vi "Vol-RPM_Tuning.vi"() -> ()   [LabVIEW 2014]
uses:
  LabView/PXI_Interface/AnalogInput/AnalogInput.lvclass
  Classes/DataLogger/Data Logger.lvclass
  <vilib>/Platform/TimedLoop/XDataNode/timing_clust.ctl
  <vilib>/Platform/TimedLoop/XDataNode/nitl_modes.ctl
  <vilib>/Platform/TimedLoop/XDataNode/wakeup.ctl
  <vilib>/FPGAPlugInAG/PXI-7842R/niLvFpga_Open_PXI-7842R.vi
  <vilib>/rvi/interface/common/dynamic/niFpgaDynamicAddResources.vi
  <vilib>/FPGAPlugInAG/Dynamic/niLvFpga_Reset_Dynamic.vi
  <vilib>/FPGAPlugInAG/Dynamic/niLvFpga_Run_Dynamic.vi
  <vilib>/Utility/error.llb/Error Cluster From Error Code.vi
  <vilib>/rvi/errors/niLvFpgaAdjustHostInterfaceError.vi
  <vilib>/addons/control/pid/pid.llb/PID Control Input Filter (DBL).vi
  <vilib>/addons/control/pid/pid.llb/PID Advanced (DBL).vi
  <vilib>/addons/control/pid/pid.llb/PID Output Rate Limiter (DBL).vi
  <vilib>/rvi/interface/nirviOpenFPGA/nirviOpenFPGA.xnode
  FPGA Bitfiles/CAlex2_FPGATarget2_MotorControl_XW+iUkbXN4U.lvbitx
  FPGA2 VIs/MotorControl_PWM+AO.vi
  <vilib>/rvi/interface/nirviMethod/nirviMethod.xnode
  <vilib>/rvi/interface/nirviReadWriteControl/nirviReadWriteControl.xnode
  <vilib>/Platform/TimedLoop/XDataNode/XDataNode.xnode
  <vilib>/Platform/TimedLoop/XDataNode/XDNodeRunTimeDep.lvlib
  <vilib>/rvi/interface/Simulation/niFpgaSimulationCallBeginRW.vi
  <vilib>/addons/control/pid/NI_PID_pid.lvlib
  Classes/MotorControl/MotorControl.lvclass
  NiFpgaLv.dll
panel:
  out "Force (N)":dbl
  in  "Enum":enum16{"1", "2", "3", "4", "5", "6", "7", "8"}(ring)
  in  "Vfb":i32=8
  out "Current(A)":dbl
  in  "Vrpm":i32=9
  out "Speed(rpm)":dbl
  in  "File Name":string
  in  "End":dbl
  in  "Begin":dbl
  in  "Start":bool
  in  "Step":dbl
  in  "Duration":dbl
  out "Current":cluster{"output":dbl}(graph)
  in  "RateLimiter":dbl=1.0 format="%.2f"
  in  "PID":bool=TRUE
  in  "Manual AO":dbl format="%.2f"
  out "Angular Rates (RPM)":dbl[](array[numeric])
  in  "AO":dbl[](array[numeric])
  in  "Zero":bool
  out "Speed":T1(graph)
  in  "setpoint":dbl format="%.2f"
  in  "reinitialize? (F)":bool
  in  "PID gains":T2={"proportional gain (Kc)"=1.0, "integral time (Ti, min)"=0.01, "derivative time (Td, min)"=0.0} {"derivative time (Td, min)" format="%.5f"; "integral time (Ti, min)" format="%.5f"; "proportional gain (Kc)" format="%.5f"}
  in  "output range":cluster{"output high":dbl, "output low":dbl}={"output high"=5.0, "output low"=-5.0} {"output low" format="%.2f"; "output high" format="%.2f"}
  in  "AO Channel":enum16{"1", "2", "3", "4", "5", "6", "7", "8"}(ring)
  in  "Encoder Channel":T3(ring)
  out "AO Value":dbl[](array[numeric]) format="%.3f"
  in  "stop":bool
  out "Angles (deg)":dbl[](array[numeric])
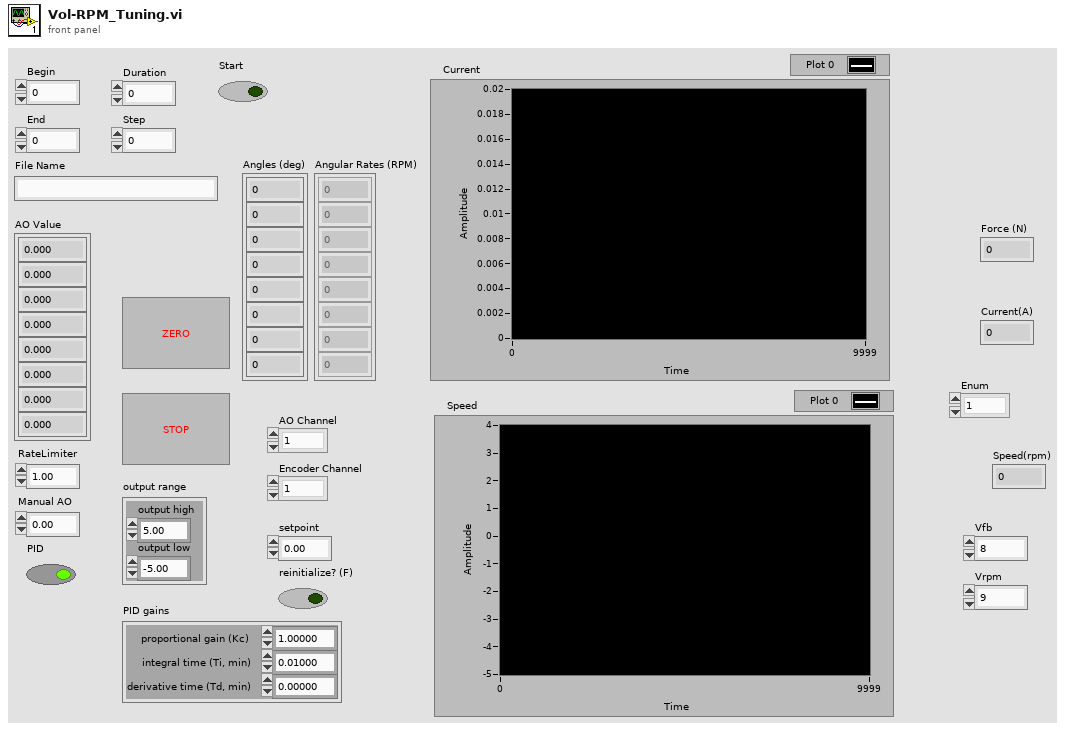
[diagram p1: front panel]
types:
  T1 = cluster{"setpoint":dbl, "output":dbl, "Speed(rpm)":dbl}
  T2 = cluster{"proportional gain (Kc)":dbl, "integral time (Ti, min)":dbl, "derivative time (Td, min)":dbl}
  T3 = enum16{"1", "2", "3", "4", "5", "6", "7", "8", "Vfb"}
  T4 = typedef "XDNodeRunTimeDep.lvlib/timing_clust.ctl" = cluster{"Expected End [f-1]":u64, "Actual End [f-1]":u64, "Finished Late? [f-1]":bool, "Expected End [i-1]":u64, "Actual End [i-1]":u64, "Finished Late? [i-1]":bool, "Expected Start [i]":u64, "Actual Start [i]":u64, "Expected Start [f]":u64, "Actual Start [f]":u64, "Source Name":string, "Structure Name":string, "Period":i64, "Deadline":i64, "Offset":i64, "Start":i64, "Priority":i32, "Timeout":i32, "Mode":T5, "Wakeup Reason":T6, "Error":errorcluster, "Source Type":string, "Secondary Source Type":string, "Global End Time":u64, "Global Start Time":u64, "Frame Duration":u64, "Iteration Duration":u64, "Assigned CPU":i32, "I/O Scan Engine Mode":u32}
  T5 = typedef "XDNodeRunTimeDep.lvlib/nitl_modes.ctl" = enum32{"No Change", "Process missed periods, maintain original phase", "Discard missed periods, maintain original phase", "Process missed periods, ignore original phase", "Discard missed periods, ignore original phase"}
  T6 = typedef "XDNodeRunTimeDep.lvlib/wakeup.ctl" = enum32{"Normal", "Aborted", "Asynchronous wakeup", "Timing source error", "Timed loop error", "Timeout"}
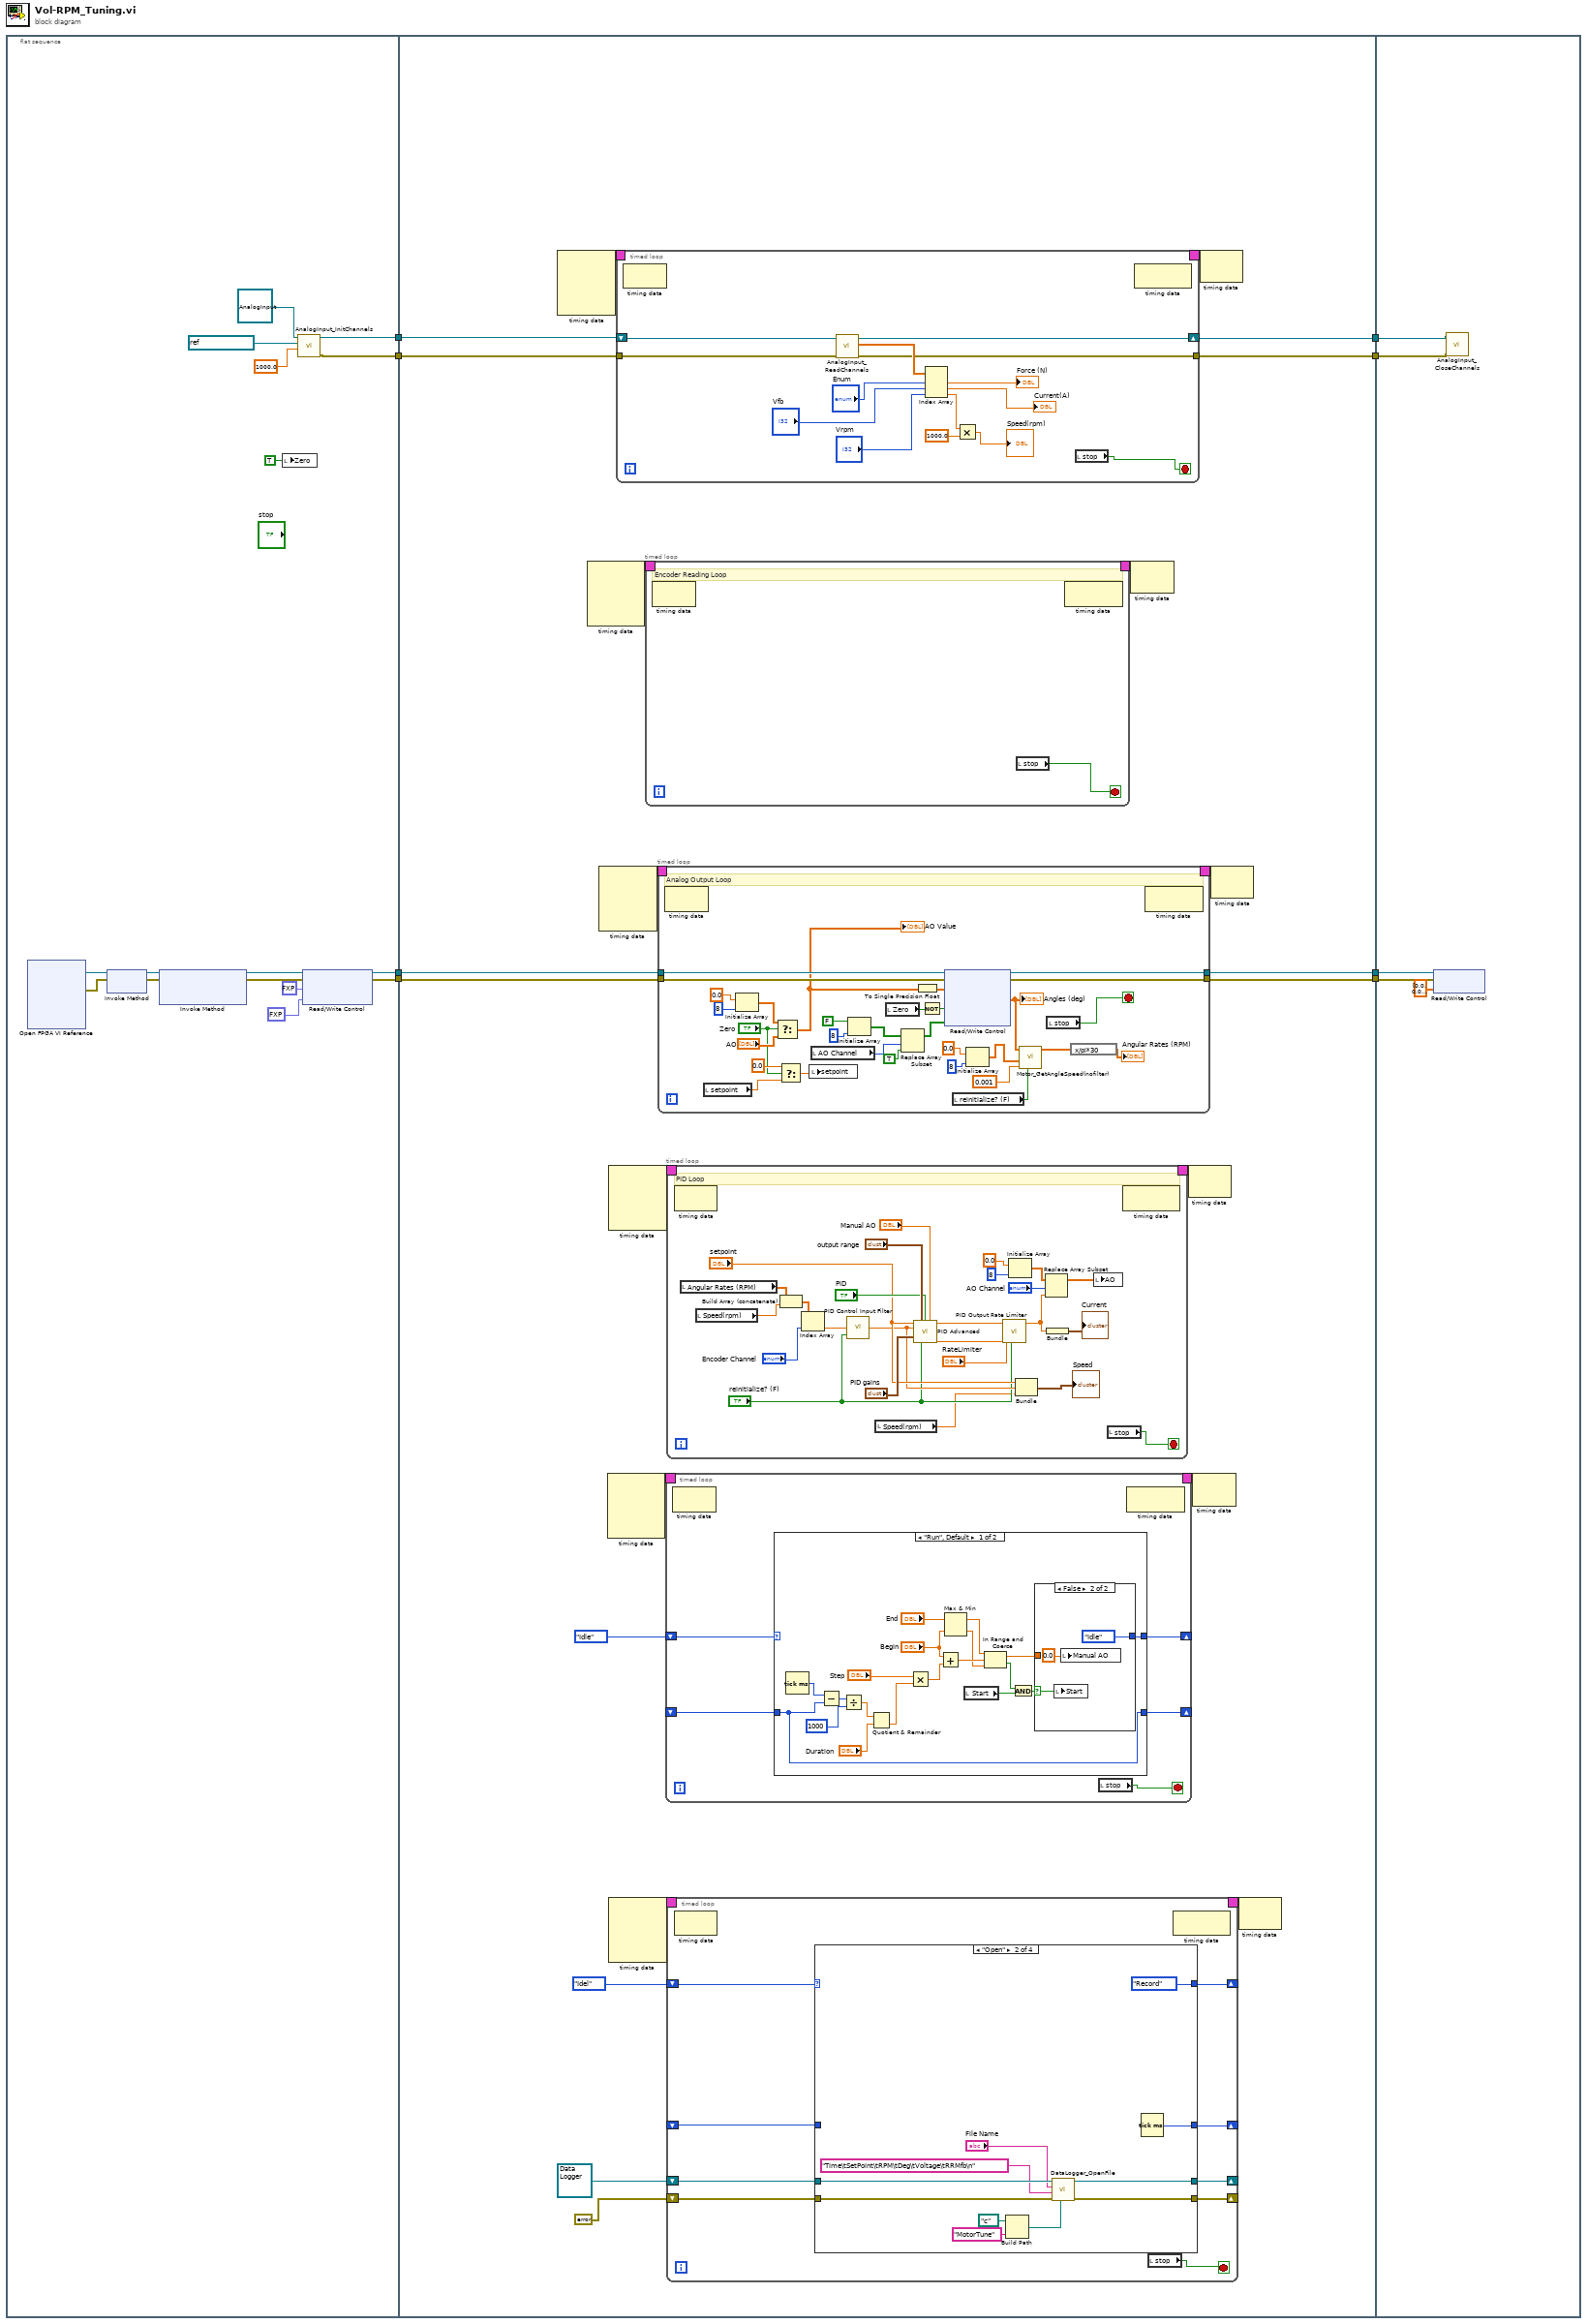
[diagram p0: block diagram]
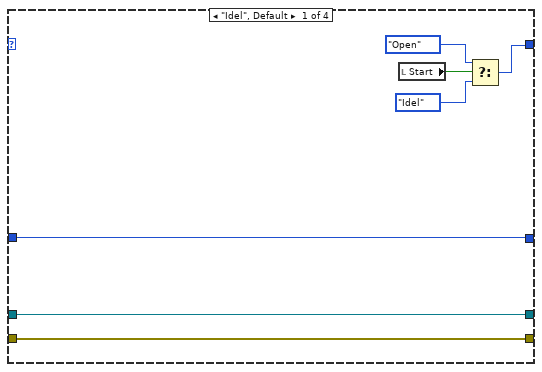
[diagram p2: hidden frame]
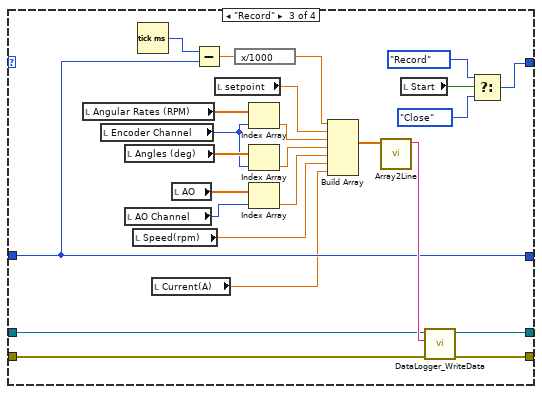
[diagram p3: hidden frame]
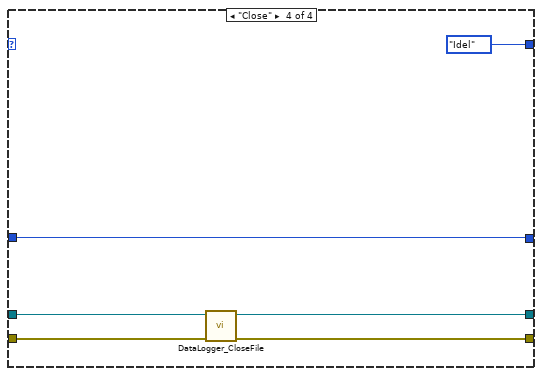
[diagram p4: hidden frame]
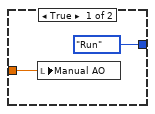
[diagram p5: hidden frame]
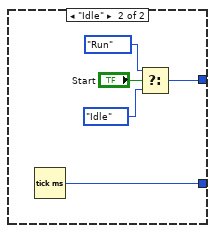
[diagram p6: hidden frame]
diagram:
  n1 = flat-sequence {
    tunnel: [w17] -> w8
    tunnel: [w16] -> w7
    tunnel: [w12] -> w2
    tunnel: [w11] -> w1
    tunnel: w8 -> [w44]
    tunnel: w7 -> [w43]
    tunnel: [w42] -> w6
    tunnel: [w41] -> w5
    tunnel: [w28] -> w4
    tunnel: [w27] -> w3
    tunnel: w2 -> [w26]
    tunnel: w1 -> [w25]
    tunnel: w6 -> [w239]
    tunnel: w5 -> [w240]
    tunnel: w4 -> [w237]
    tunnel: w3 -> [w236]
    frame #0 {
      n2 = xnode "Open FPGA VI Reference"() -> ("FPGA VI Reference Out"=w24:refnum<k20>, "error out"=w23:errorcluster)  [unwired: 2 in]
      n3 = xnode "Invoke Method"("FPGA VI Reference In"=w24, "error in"=w23) -> ("FPGA VI Reference Out"=w22:refnum<k20>, "error out"=w21:errorcluster)
      n4 = xnode "Invoke Method"("FPGA VI Reference In"=w22, "error in"=w21) -> ("FPGA VI Reference Out"=w19:refnum<k20>, "error out"=w18:errorcluster)  [unwired: 1 in]
      n5 = local write "Zero"(TRUE ("Zero")) -> ()
      n6 = call "AnalogInput_InitChannels.vi"("SampFreq"=1000.0, "Analog Input Channels"=refnum<k21> "TuningTask", "AnalogInput in"=refnum<class "AnalogInput.lvclass"> refnum ("AnalogInput")) -> ("error out"=w11:errorcluster, "AnalogInput out"=w12:refnum<class "AnalogInput.lvclass">)  [unwired: 7 in]
      n7 = xnode "Read/Write Control"("FPGA VI Reference In"=w19, "error in"=w18, "PWM (Hz/A)"=fxp<+/-,32,16> 1.0, "EncoderCount"=fxp<+,16,16> 500.0) -> ("FPGA VI Reference Out"=w17:refnum<k20>, "error out"=w16:errorcluster)
    }
    frame #1 {
      n8 = node-c288() -> (w30:T4)  [unwired: 4 in]
      n9 = node-c288() -> (w48:T4)  [unwired: 4 in]
      n10 = node-c288() -> (w46:T4)  [unwired: 4 in]
      n11 = node-c288() -> (w38:T4)  [unwired: 4 in]
      n12 = node-c288() -> (w40:T4)  [unwired: 4 in]
      n13 = node-c288() -> (w35:T4)  [unwired: 4 in]
      n14 = timed-loop {
        timing: w30 -> [_]
        timing-out: [_] -> w29
        shift-right: [w61] -> w28
        shift-left: w26 -> [w62]
        tunnel: w25 -> [w58]
        tunnel: [w57] -> w27
        stop <- w55 stop-if-true
        n15 = node-c288() -> ()  [unwired: 1 in, 1 out]
        n16 = call "AnalogInput_ReadChannels.vi"("error in (no error)"=w58, "AnalogInput in"=w62) -> ("error out"=w57:errorcluster, "AI readings"=w60:dbl[], "AnalogInput out"=w61:refnum<class "AnalogInput.lvclass">)  [unwired: 7 in]
        n17 = Index Array(array=w60, index #1="Enum", index #2="Vfb", index #3="Vrpm") -> (element #1=→"Force (N)":dbl, element #2=→"Current(A)":dbl, element #3=w51:dbl)
        n18 = Multiply(x=w51, y=1000.0) -> (x*y=→"Speed(rpm)":dbl)
        n19 = local read "stop"() -> (w55:bool)
        n20 = node-c288() -> ()  [unwired: 1 in, 1 out]
      }
      n21 = timed-loop {
        timing: w48 -> [_]
        timing-out: [_] -> w47
        stop <- w231 stop-if-true
        # "Encoder Reading Loop"
        n22 = node-c288() -> ()  [unwired: 1 in, 1 out]
        n23 = local read "stop"() -> (w231:bool)
        n24 = node-c288() -> ()  [unwired: 1 in, 1 out]
      }
      n25 = timed-loop {
        timing: w46 -> [_]
        timing-out: [_] -> w45
        tunnel: w44 -> [w226]
        tunnel: w43 -> [w225]
        tunnel: [w224] -> w41
        tunnel: [w223] -> w42
        stop <- w212 stop-if-true
        # "Analog Output Loop"
        n26 = node-c288() -> ()  [unwired: 1 in, 1 out]
        n27 = local read "setpoint"() -> (w214:dbl)
        n28 = Initialize Array(0.0 ("element"), 8 ("dimension size")) -> (w220:dbl[])
        n29 = Select(t=w220, s="Zero", f="AO") -> (s? t:f=w217:dbl[])
        "AO Value" <- w217
        n30 = Select(t=0.0 ("element"), s="Zero", f=w214) -> (s? t:f=w216:dbl)
        n31 = local write "setpoint"(w216) -> ()
        n32 = local read "AO Channel"() -> (w206:enum16{"1", "2", "3", "4", "5", "6", "7", "8"})
        n33 = Initialize Array(FALSE ("Zero"), 8 ("dimension size")) -> (w207:bool[])
        n34 = local read "Zero"() -> (w211:bool)
        n35 = Replace Array Subset(array=w207, new element=TRUE ("new element/subarray"), index=w206) -> (w204:bool[])
        n36 = To Single Precision Float(number=w217) -> (single precision float=w218:sgl[])
        n37 = Not(x=w211) -> (.not. x?=w210:bool)
        n38 = xnode "Read/Write Control"("FPGA VI Reference In"=w226, "error in"=w225, "AmpCmd"=w218, "EnableMaster"=w210, "Enable"=w204) -> ("FPGA VI Reference Out"=w224:refnum<k20>, "error out"=w223:errorcluster, "EncdAngle"=w203:sgl[])
        "Angles (deg)" <- w203
        n39 = local read "reinitialize? (F)"() -> (w198:bool)
        n40 = Initialize Array(0.0 ("element"), 8 ("dimension size")) -> (w201:dbl[])
        n41 = call "Motor_GetAngleSpeed(nofilter).vi"("initialize"=w198, "dt"=0.001, "Initial Condition"=w201, "Angles"=w203) -> ("AngularSpeed"=w197:dbl[])  [unwired: 7 in]
        n42 = local read "stop"() -> (w212:bool)
        n43 = expression code="x/pi*30"(w197) -> (→"Angular Rates (RPM)":dbl[])
        n44 = node-c288() -> ()  [unwired: 1 in, 1 out]
      }
      n45 = timed-loop {
        timing: w38 -> [_]
        timing-out: [_] -> w37
        shift-right: [w130] -> _
        shift-left: enum16{"Run", "Idle"}."Idle" -> [w133]
        shift-right: [w132] -> _
        shift-left: _ -> [w131]
        stop <- w129 stop-if-true
        n46 = node-c288() -> ()  [unwired: 1 in, 1 out]
        n47 = case shown="\"Run\", Default" w133 {
          tunnel: [w137 w162] -> w132
          tunnel: w131 -> [w137 _]
          tunnel: [w135 w160] -> w130
          frame "Run", Default {
            n48 = Tick Count (ms)() -> (millisecond timer value=w152:u32)
            n49 = Subtract(x=w152, y=w137) -> (x-y=w151:u32)
            n50 = Divide(x=w151, y=u32 1000) -> (x/y=w148:dbl)
            n51 = Quotient & Remainder(x=w148, y="Duration") -> (floor(x/y)=w146:dbl)  [unwired: 1 out]
            n52 = Multiply(x="Step", y=w146) -> (x*y=w145:dbl)
            n53 = Add(x="Begin", y=w145) -> (x+y=w144:dbl)
            n54 = Max & Min(x="End", y="Begin") -> (max(x,y)=w141:dbl, min(x,y)=w140:dbl)
            n55 = local read "Start"() -> (w139:bool)
            n56 = In Range and Coerce(upper limit=w141, x=w144, lower limit=w140) -> (coerced(x)=w134:dbl, In Range?=w138:bool)
            n57 = And(x=w138, y=w139) -> (x .and. y?=w136:bool)
            n58 = case shown="False" w136 {
              selector: w136 -> [_ w155]
              tunnel: [enum16{"Run", "Idle"}."Run" enum16{"Run", "Idle"}."Idle"] -> w135
              tunnel: w134 -> [w153 _]
              frame True {
                n59 = local write "Manual AO"(w153) -> ()
              }
              frame False {
                n60 = local write "Start"(w155) -> ()
                n61 = local write "Manual AO"(0.0 ("f")) -> ()
              }
            }
          }
          frame "Idle" {
            n62 = Tick Count (ms)() -> (millisecond timer value=w162:u32)
            n63 = Select(t=enum16{"Run", "Idle"}."Run", s="Start", f=enum16{"Run", "Idle"}."Idle") -> (s? t:f=w160:enum16{"Run", "Idle"})
          }
        }
        n64 = local read "stop"() -> (w129:bool)
        n65 = node-c288() -> ()  [unwired: 1 in, 1 out]
      }
      n66 = timed-loop {
        timing: w40 -> [_]
        timing-out: [_] -> w39
        stop <- w171 stop-if-true
        # "PID Loop"
        n67 = node-c288() -> ()  [unwired: 1 in, 1 out]
        n68 = local read "Angular Rates (RPM)"() -> (w170:dbl[])
        n69 = local read "Speed(rpm)"() -> (w169:dbl)
        n70 = Build Array (concatenate)(w170, w169) -> (w168:dbl[])
        n71 = Index Array(array=w168, index="Encoder Channel") -> (element=w173:dbl)
        n72 = call-poly <vilib>:"PID Control Input Filter.vi"("reinitialize? (F)"="reinitialize? (F)", "input"=w173) -> ("output"=w174:dbl)  [unwired: 3 in]
        n73 = local read "Speed(rpm)"() -> (w167:dbl)
        n74 = call-poly <vilib>:"PID Advanced.vi"("setpoint"="setpoint", "output range"="output range", "auto? (T)"="PID", "manual control"="Manual AO", "process variable"=w174, "PID gains"="PID gains", "reinitialize? (F)"="reinitialize? (F)") -> ("output"=w180:dbl, "dt out (s)"=w179:dbl)  [unwired: 7 in]
        n75 = call-poly <vilib>:"PID Output Rate Limiter.vi"("reinitialize? (F)"="reinitialize? (F)", "dt (s)"=w179, "output rate (EGU/min)"="RateLimiter", "input (controller output)"=w180) -> ("output"=w175:dbl)  [unwired: 4 in, 1 out]
        n76 = Initialize Array(0.0 ("element"), 8 ("dimension size")) -> (w188:dbl[])
        n77 = Bundle("setpoint"="setpoint", "output"=w174, "Speed(rpm)"=w167) -> (→"Speed":T1)  [unwired: 1 in]
        n78 = Replace Array Subset(array=w188, new element=w175, index="AO Channel") -> (w189:dbl[])
        n79 = Bundle("output"=w175) -> (→"Current":cluster{"output":dbl})  [unwired: 1 in]
        n80 = local write "AO"(w189) -> ()
        n81 = local read "stop"() -> (w171:bool)
        n82 = node-c288() -> ()  [unwired: 1 in, 1 out]
      }
      n83 = timed-loop {
        timing: w35 -> [_]
        timing-out: [_] -> w34
        shift-right: [w73] -> _
        shift-left: refnum<class "Data Logger.lvclass"> refnum ("Data Logger out") -> [w74]
        shift-right: [w72] -> _
        shift-left: errorcluster {"status"=FALSE, "code"=0, "source"=""} ("error out") -> [w71]
        shift-right: [w69] -> _
        shift-left: _ -> [w70]
        shift-right: [w68] -> _
        shift-left: enum16{"Close", "Record", "Open", "Idel"}."Idel" -> [w75]
        stop <- w67 stop-if-true
        n84 = node-c288() -> ()  [unwired: 1 in, 1 out]
        n85 = case shown="\"Open\"" w75 {
          tunnel: w74 -> [w82 w93 w105 w124]
          tunnel: [w82 w84 w118 w122] -> w73
          tunnel: [w81 w83 w117 w121] -> w72
          tunnel: w71 -> [w81 w92 w104 w123]
          tunnel: w70 -> [w76 _ w102 w120]
          tunnel: [w76 w89 w102 w120] -> w69
          tunnel: [w79 enum16{"Close", "Record", "Open", "Idel"}."Record" w98 enum16{"Close", "Record", "Open", "Idel"}."Idel"] -> w68
          frame "Idel", Default {
            n86 = local read "Start"() -> (w80:bool)
            n87 = Select(t=enum16{"Close", "Record", "Open", "Idel"}."Open", s=w80, f=enum16{"Close", "Record", "Open", "Idel"}."Idel") -> (s? t:f=w79:enum16{"Close", "Record", "Open", "Idel"})
          }
          frame "Open" {
            n88 = Build Path(base path=path "c:/", name or relative path="MotorTune" ("ProjectFolder")) -> (appended path=w86:path)
            n89 = call "DataLogger_OpenFile.vi"("base path"=w86, "error in (no error)"=w92, "Header"="Time\tSetPoint\tRPM\tDeg\tVoltage\tRRMfb\n", "File Name"="File Name", "Data Logger in"=w93) -> ("error out"=w83:errorcluster, "Data Logger out"=w84:refnum<class "Data Logger.lvclass">)  [unwired: 5 in]
            n90 = Tick Count (ms)() -> (millisecond timer value=w89:u32)
          }
          frame "Record" {
            n91 = local read "Angular Rates (RPM)"() -> (w116:dbl[])
            n92 = local read "Encoder Channel"() -> (w114:T3)
            n93 = local read "Angles (deg)"() -> (w115:dbl[])
            n94 = local read "AO Channel"() -> (w113:enum16{"1", "2", "3", "4", "5", "6", "7", "8"})
            n95 = local read "Speed(rpm)"() -> (w95:dbl)
            n96 = Tick Count (ms)() -> (millisecond timer value=w103:u32)
            n97 = local read "Current(A)"() -> (w94:dbl)
            n98 = local read "AO"() -> (w112:dbl[])
            n99 = Subtract(x=w103, y=w102) -> (x-y=w97:dbl)
            n100 = local read "setpoint"() -> (w111:dbl)
            n101 = expression code="x/1000"(w97) -> (w96:dbl)
            n102 = Index Array(array=w116, index=w114) -> (element=w110:dbl)
            n103 = Index Array(array=w115, index=w114) -> (element=w109:dbl)
            n104 = Index Array(array=w112, index=w113) -> (element=w108:dbl)
            n105 = Build Array(w96, w111, w110, w109, w108, w95, w94) -> (w107:dbl[])
            n106 = call "Array2Line.vi"("Data"=w107) -> ("String"=w106:string)  [unwired: 10 in]
            n107 = local read "Start"() -> (w101:bool)
            n108 = call "DataLogger_WriteData.vi"("error in (no error)"=w104, "New line"=w106, "Data Logger in"=w105) -> ("error out"=w117:errorcluster, "Data Logger out"=w118:refnum<class "Data Logger.lvclass">)  [unwired: 7 in]
            n109 = Select(t=enum16{"Close", "Record", "Open", "Idel"}."Record", s=w101, f=enum16{"Close", "Record", "Open", "Idel"}."Close") -> (s? t:f=w98:enum16{"Close", "Record", "Open", "Idel"})
          }
          frame "Close" {
            n110 = call "DataLogger_CloseFile.vi"("error in (no error)"=w123, "Data Logger in"=w124) -> ("error out"=w121:errorcluster, "Data Logger out"=w122:refnum<class "Data Logger.lvclass">)  [unwired: 8 in]
          }
        }
        n111 = local read "stop"() -> (w67:bool)
        n112 = node-c288() -> ()  [unwired: 1 in, 1 out]
      }
      n113 = node-c288(w47) -> ()  [unwired: 1 out]
      n114 = node-c288(w39) -> ()  [unwired: 1 out]
      n115 = node-c288(w37) -> ()  [unwired: 1 out]
      n116 = node-c288(w29) -> ()  [unwired: 1 out]
      n117 = node-c288(w45) -> ()  [unwired: 1 out]
      n118 = node-c288(w34) -> ()  [unwired: 1 out]
    }
    frame #2 {
      n119 = xnode "Read/Write Control"("FPGA VI Reference In"=w240, "error in"=w239, "AmpCmd"=sgl[] [0.0, 0.0, 0.0, 0.0, 0.0, 0.0, 0.0, 0.0] ("AO_Value")) -> ()  [unwired: 2 out]
      n120 = call "AnalogInput_CloseChannels.vi"("error in (no error)"=w236, "AI"=w237) -> ()  [unwired: 9 in, 1 out]
    }
  }
